vi "Syntax Check.vi"(5 "Denominator":dbl[](array[numeric]) format="%.2f", 6 "Numerator":dbl[](array[numeric])=[1.0] format="%.2f") -> (0 "error":i32, 1 "gain":dbl format="%.2f", 2 "Denominator new":dbl[](array[numeric]) format="%.2f", 3 "Numerator new IC":dbl[](array[numeric]) format="%.2f", 4 "Numerator new":dbl[](array[numeric]) format="%.2f")   [LabVIEW 2017, in "NI_AdvCtrl_continuous linear.lvlib"]
doc: "LabVIEW no longer supports this VI. You can obtain similar functionality by installing the LabVIEW Simulation Module."
uses:
  <vilib>/addons/control/advanced/NI_AdvCtrl_continuous linear.lvlib
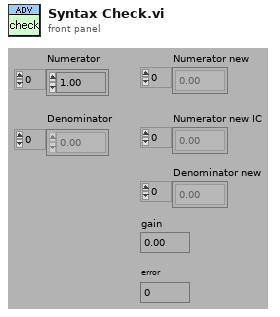
[diagram p1: front panel]
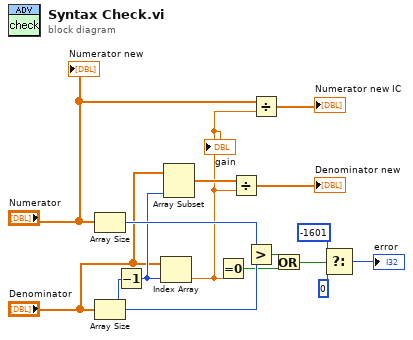
[diagram p0: block diagram]
diagram:
  n1 = Array Size(array="Numerator") -> (size(s)=w15:i32)
  n2 = Array Size(array="Denominator") -> (size(s)=w14:i32)
  n3 = Decrement(x=w14) -> (x-1=w13:i32)
  n4 = Index Array(array="Denominator", index=w13) -> (element=w7:dbl)
  "gain" <- w7
  n5 = Array Subset(array="Denominator", length=w13) -> (w11:dbl[])  [unwired: 1 in]
  n6 = Equal To 0?(x=w7) -> (x = 0?=w10:bool)
  n7 = Divide(x=w11, y=w7) -> (x/y=→"Denominator new":dbl[])
  n8 = Greater?(x=w15, y=w14) -> (0:w8:bool)
  n9 = Divide(x="Numerator", y=w7) -> (x/y=→"Numerator new IC":dbl[])
  n10 = Or(x=w8, y=w10) -> (x .or. y?=w2:bool)
  n11 = Select(t=-1601 ("error"), s=w2, f=0 ("error")) -> (s? t:f=→"error":i32)
  "Numerator new" <- "Numerator"
